vi "get_raw_data.vi"(8 "error in (no error)":errorcluster, 11 "MeasurementResult in":refnum<class "MeasurementResult.lvclass">) -> (0 "error out":errorcluster, 2 "raw_data":u16[][](array[numeric]), 3 "MeasurementResult out":refnum<class "MeasurementResult.lvclass">)   [LabVIEW 2017, in "MeasurementResult.lvclass"]
uses:
  MeasurementResult.lvclass
  MeasurementResult.lvclass/MeasurementResult.ctl
panel:
  # "2d array of u16"
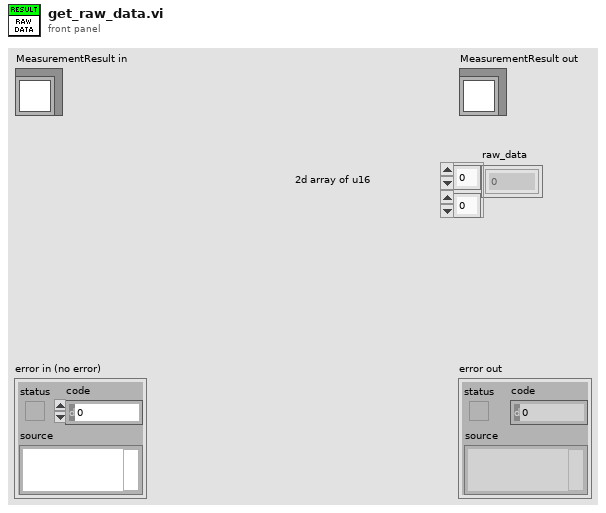
[diagram p1: front panel]
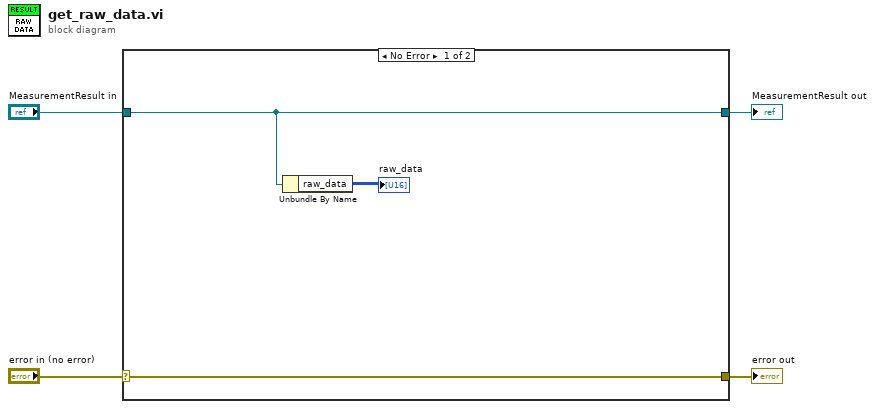
[diagram p0: block diagram]
diagram:
  n1 = case shown="No Error" "error in (no error)" {
    selector: "error in (no error)" -> [w7 w9]
    tunnel: [w7 w9] -> w3
    tunnel: [w6 w8] -> w1
    tunnel: "MeasurementResult in" -> [w6 w8]
    frame No Error {
      n2 = Unbundle By Name(w6) -> ("raw_data"=→"raw_data":u16[][])
    }
    frame Error {
    }
  }
  "error out" <- w3
  "MeasurementResult out" <- w1
